vi "20151005 Save transition sample.vi"(8 "error in":errorcluster, 10 "Data":T1[](array[typedef]), 11 "Collect data save pos":path) -> (0 "error out":errorcluster)   [LabVIEW 2013]
uses:
  Q-neural/controls/Sample set.ctl
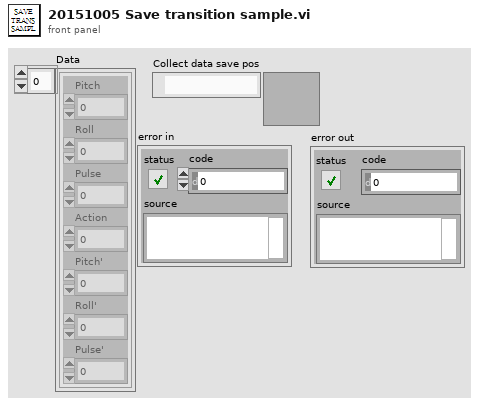
[diagram p1: front panel]
types:
  T1 = typedef "Sample set.ctl" = cluster{"Pitch":dbl, "Roll":dbl, "Pulse":dbl, "Action":dbl, "Pitch'":dbl, "Roll'":dbl, "Pulse'":dbl}
  T2 = enum16{"open", "replace", "create", "open or create", "replace or create", "replace or create with confirmation"}
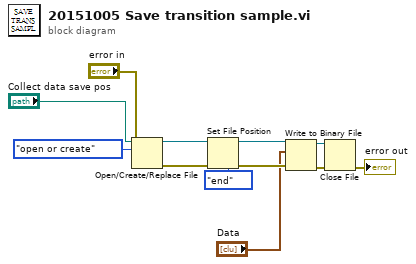
[diagram p0: block diagram]
diagram:
  n1 = Open/Create/Replace File(file path (use dialog)="Collect data save pos", error in="error in", operation (0:open)=T2."open or create") -> (refnum out=w7:refnum<file>, error out=w9:errorcluster)  [unwired: 3 in, 1 out]
  n2 = Set File Position(refnum=w7, from (0:start)=enum16{"start", "end", "current"}."end", error in=w9) -> (refnum out=w6:refnum<file>, error out=w8:errorcluster)  [unwired: 1 in]
  n3 = Write to Binary File(file (use dialog)=w6, data="Data", error in=w8) -> (refnum out=w10:refnum<file>, error out=w12:errorcluster)  [unwired: 3 in, 1 out]
  n4 = Close File(refnum=w10, error in=w12) -> (error out=→"error out":errorcluster)  [unwired: 1 out]
